vi "Weather_Client.vi"() -> ()   [LabVIEW 2024]
uses:
  <vilib>/express/express arith-compare/Formula/XNode/ExpressFormulaBlockNode.xnode
  <vilib>/httpClient/LabVIEWHTTPClient.lvlib
panel:
  in  "stop":bool
  out "Cloud Coverage [%]":dbl
  out "Slide":u8(slide) scale=0.0..100.0
  out "Wind Direction":dbl(knob) scale=0.0..312.0
  out "Wind Speed [m/s]":dbl(knob) scale=0.0..10.0
  out "Wind":T1
  out "Country":string
  out "Sunset (24h)":string
  out "Sunrise (24h)":string
  out "Current Time":timestamp format="%<%I:%M %p\n%x>T"
  out "Humidity Meter":dbl(knob) scale=0.0..100.0
  out "Humidity (%)":i32
  out "Pressure [hPa]":dbl
  out "Max Temp":dbl
  out "Min Temp":dbl
  out "Feels Like":dbl
  out "Thermometer":dbl(slide) scale=0.0..50.0
  in  "Select [°C/°F/K]":enum16{"Celcius", "Farenheit", "Kelvin"}(ring)
  out "Current Temp":dbl
  out "Status":cluster{"Sky":string, "Description":string}[](array[cluster])
  out "Coordinates":cluster{"Logitude":dbl, "Latitude":dbl}
  out "Visibility [km]":i32
  out "City Chosen":string
  in  "Enter City Name":string
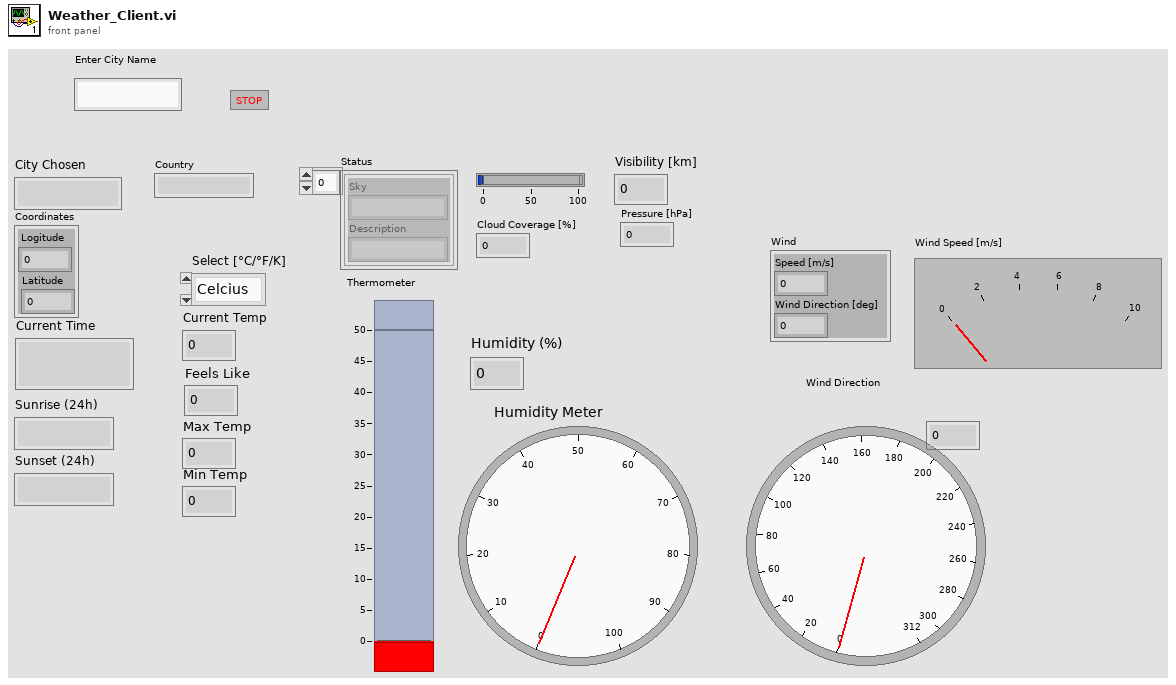
[diagram p1: front panel]
types:
  T1 = cluster{"Speed [m/s]":dbl, "Wind Direction [deg]":dbl}
  T2 = cluster{"sunrise":dbl, "sunset":dbl, "country":string}
  T3 = cluster{"temp":dbl, "feels_like":dbl, "temp_min":dbl, "temp_max":dbl, "pressure":dbl, "humidity":dbl}
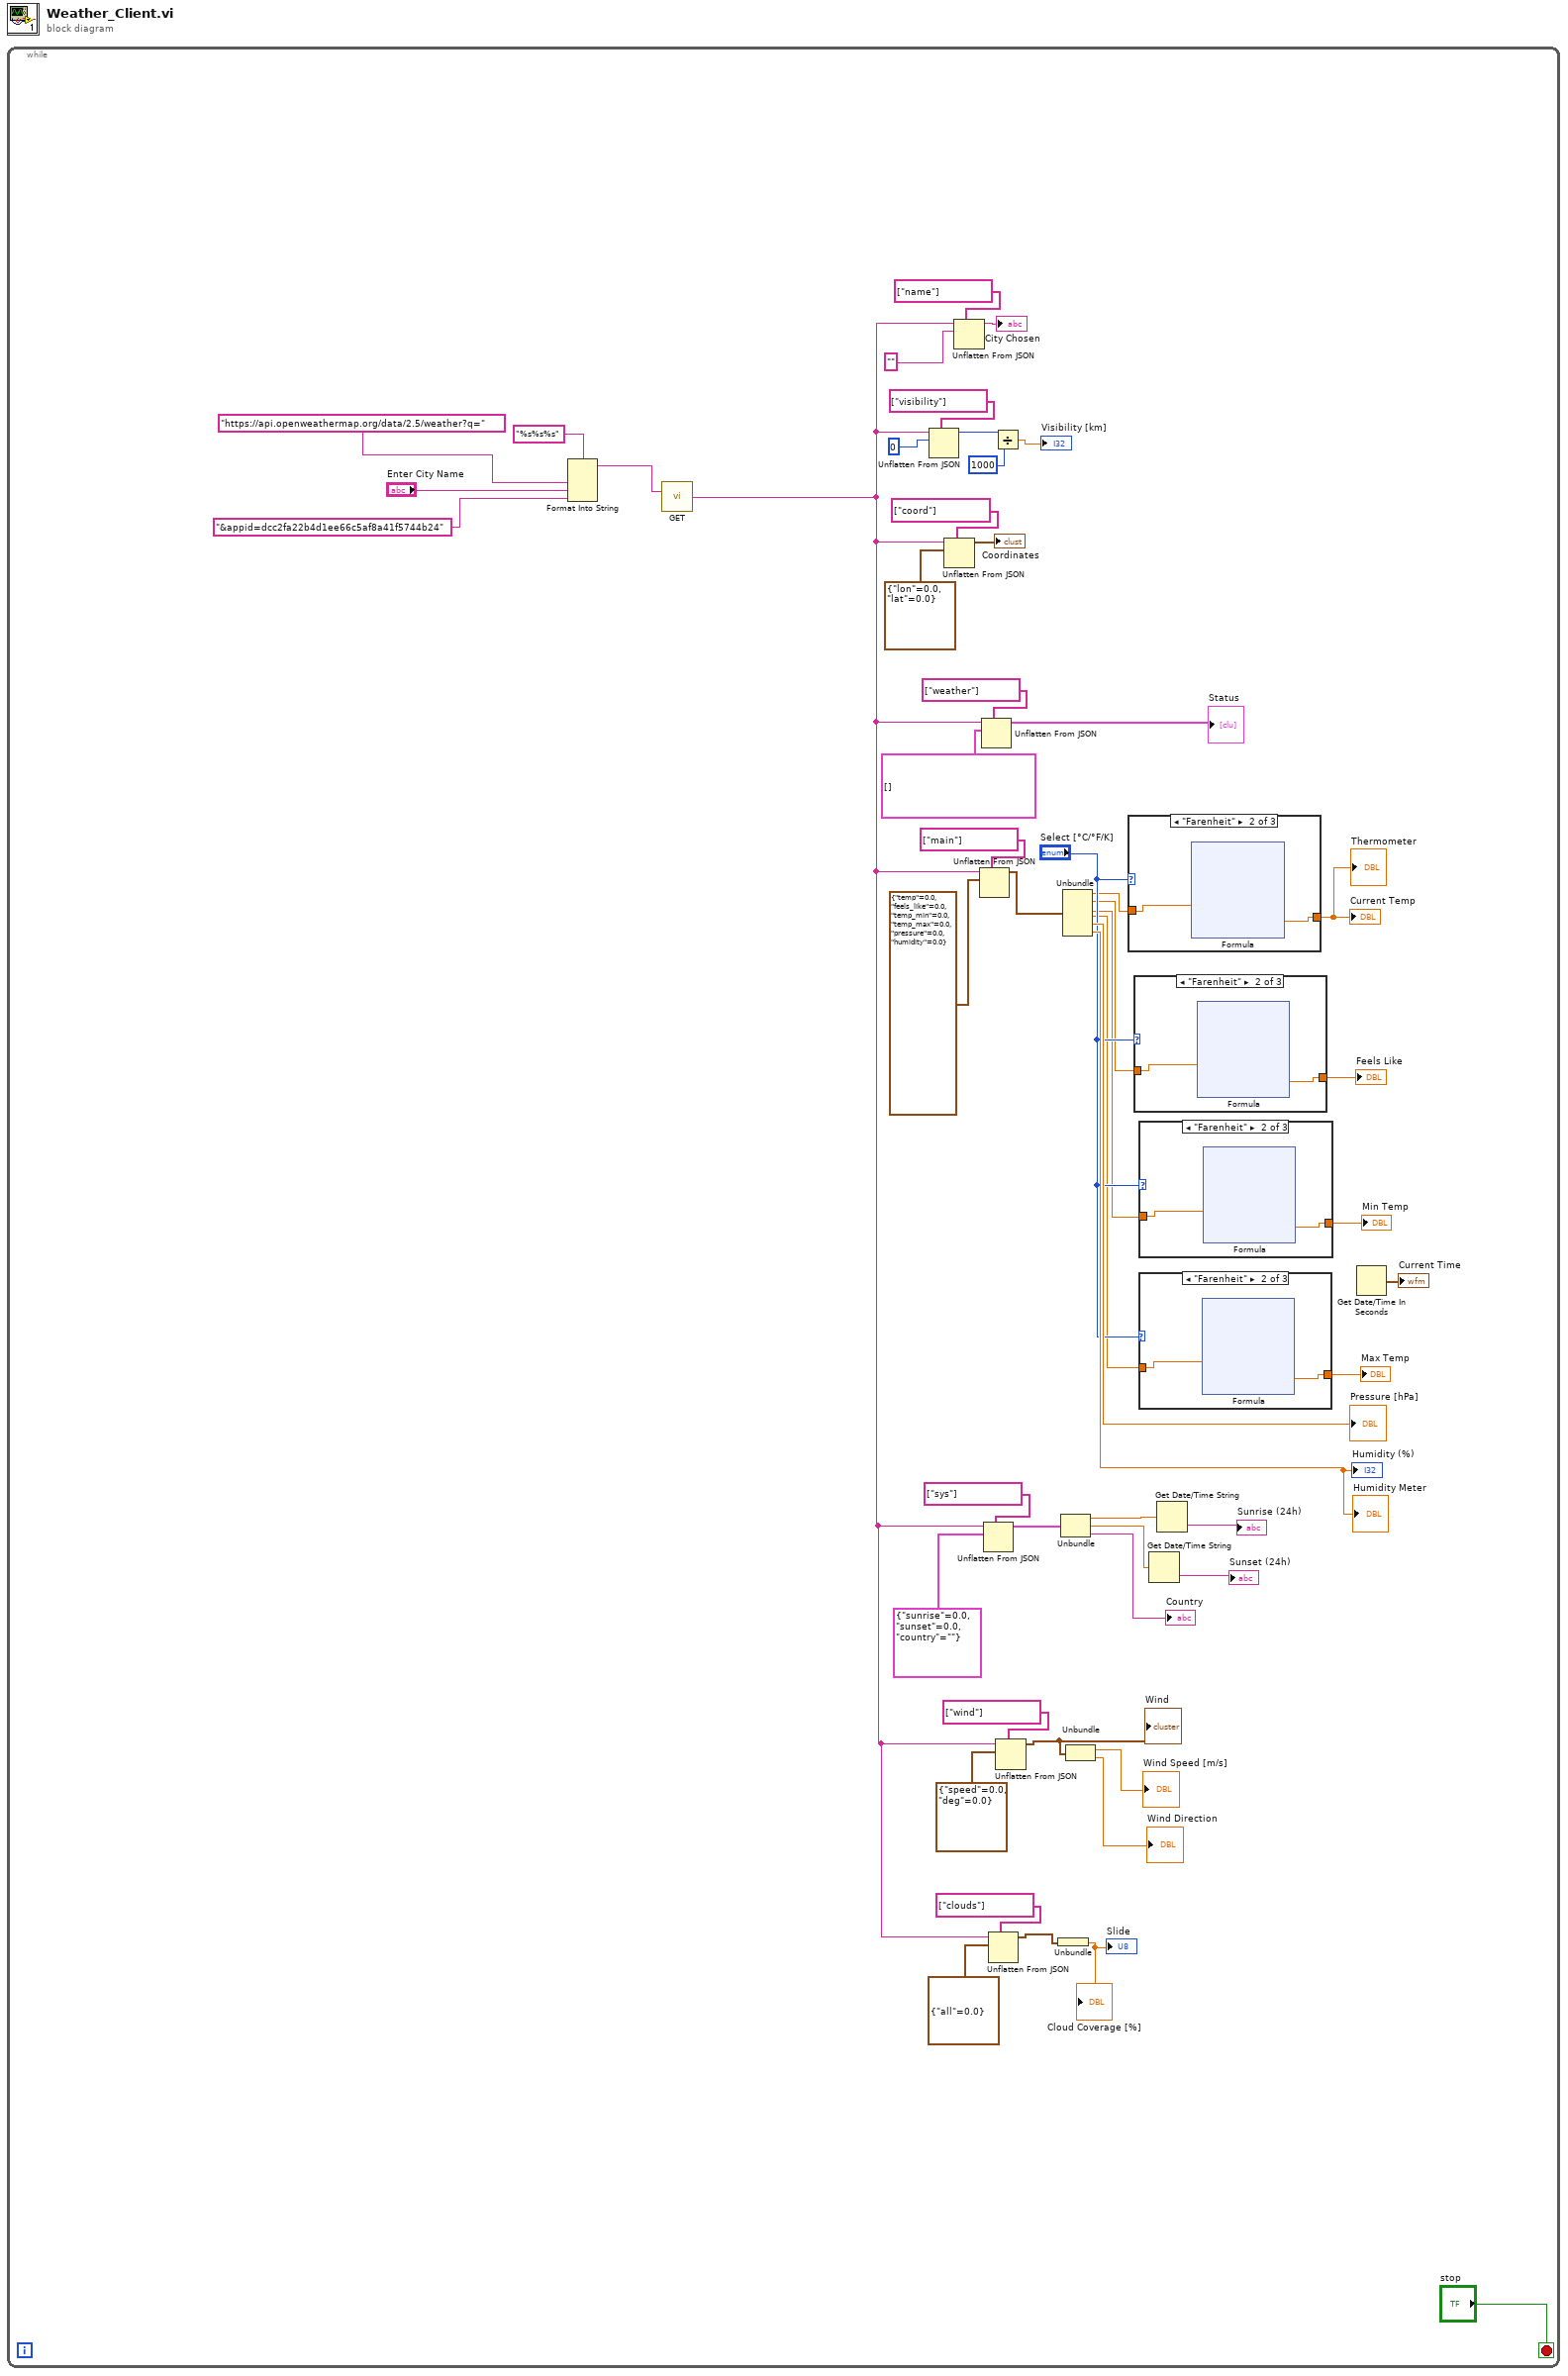
[diagram p0: block diagram]
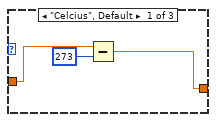
[diagram p2: hidden frame]
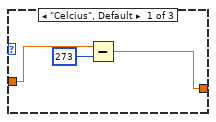
[diagram p4: hidden frame]
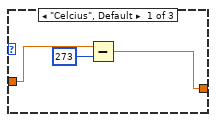
[diagram p6: hidden frame]
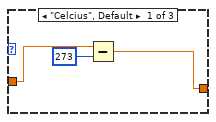
[diagram p8: hidden frame]
diagram:
  n1 = while {
    stop <- "stop" stop-if-true
    n2 = Format Into String(format string="%s%s%s", "https://api.openweathermap.org/data/2.5/weather?q=" ("input 1"), "Enter City Name", "&appid=dcc2fa22b4d1ee66c5af8a41f5744b24" ("input 3")) -> (resulting string=w22:string)  [unwired: 2 in, 1 out]
    n3 = call <vilib>:"GET.vi"("url"=w22) -> ("body"=w50:string)  [unwired: 11 in, 3 out]
    n4 = Unflatten From JSON(path=string[] ["visibility"], JSON string=w50, type and defaults=0 ("y")) -> (value=w24:i32)  [unwired: 4 in, 1 out]
    n5 = Unflatten From JSON(path=string[] ["coord"], JSON string=w50, type and defaults=cluster{"lon":dbl, "lat":dbl} {"lon"=0.0, "lat"=0.0}) -> (value=→"Coordinates":cluster{"lon":dbl, "lat":dbl})  [unwired: 4 in, 1 out]
    n6 = Unflatten From JSON(path=string[] ["name"], JSON string=w50, type and defaults="") -> (value=→"City Chosen":string)  [unwired: 4 in, 1 out]
    n7 = Unflatten From JSON(path=string[] ["main"], JSON string=w50, type and defaults=T3 {"temp"=0.0, "feels_like"=0.0, "temp_min"=0.0, "temp_max"=0.0, "pressure"=0.0, "humidity"=0.0}) -> (value=w30:T3)  [unwired: 4 in, 1 out]
    n8 = Unflatten From JSON(path=string[] ["weather"], JSON string=w50, type and defaults=cluster{"main":string, "description":string}[] []) -> (value=→"Status":cluster{"main":string, "description":string}[])  [unwired: 4 in, 1 out]
    n9 = Unflatten From JSON(path=string[] ["sys"], JSON string=w50, type and defaults=T2 {"sunrise"=0.0, "sunset"=0.0, "country"=""}) -> (value=w41:T2)  [unwired: 4 in, 1 out]
    n10 = Unflatten From JSON(path=string[] ["clouds"], JSON string=w50, type and defaults=cluster{"all":dbl} {"all"=0.0}) -> (value=w51:cluster{"all":dbl})  [unwired: 4 in, 1 out]
    n11 = Divide(x=w24, y=1000) -> (x/y=→"Visibility [km]":dbl)
    n12 = Unflatten From JSON(path=string[] ["wind"], JSON string=w50, type and defaults=cluster{"speed":dbl, "deg":dbl} {"speed"=0.0, "deg"=0.0}) -> (value=w47:cluster{"speed":dbl, "deg":dbl})  [unwired: 4 in, 1 out]
    "Wind" <- w47
    n13 = Unbundle(w51) -> ("all"=→"Slide" →"Cloud Coverage [%]":dbl)
    n14 = Unbundle(w41) -> ("sunrise"=w44:dbl, "sunset"=w45:dbl, "country"=→"Country":string)
    n15 = Unbundle(w30) -> ("temp"=w29:dbl, "feels_like"=w32:dbl, "temp_min"=w34:dbl, "temp_max"=w36:dbl, "pressure"=→"Pressure [hPa]":dbl, "humidity"=→"Humidity (%)" →"Humidity Meter":dbl)
    n16 = Unbundle(w47) -> ("speed"=→"Wind Speed [m/s]":dbl, "deg"=→"Wind Direction":dbl)
    n17 = case shown="\"Farenheit\"" "Select [°C/°F/K]" {
      tunnel: [w96 w99 w109] -> w28
      tunnel: w29 -> [w98 w100 w109]
      frame "Celcius", Default {
        n18 = Subtract(x=w98, y=273) -> (x-y=w96:dbl)
      }
      frame "Farenheit" {
        n19 = xnode "Formula"("X1"=w100) -> ("Result"=w99:dbl)  [unwired: 1 in, 1 out]
      }
      frame "Kelvin" {
      }
    }
    "Current Temp" <- w28
    "Thermometer" <- w28
    n20 = case shown="\"Farenheit\"" "Select [°C/°F/K]" {
      tunnel: [w82 w85 w95] -> w31
      tunnel: w32 -> [w84 w86 w95]
      frame "Celcius", Default {
        n21 = Subtract(x=w84, y=273) -> (x-y=w82:dbl)
      }
      frame "Farenheit" {
        n22 = xnode "Formula"("X1"=w86) -> ("Result"=w85:dbl)  [unwired: 1 in, 1 out]
      }
      frame "Kelvin" {
      }
    }
    "Feels Like" <- w31
    n23 = case shown="\"Farenheit\"" "Select [°C/°F/K]" {
      tunnel: [w54 w57 w67] -> w35
      tunnel: w36 -> [w56 w58 w67]
      frame "Celcius", Default {
        n24 = Subtract(x=w56, y=273) -> (x-y=w54:dbl)
      }
      frame "Farenheit" {
        n25 = xnode "Formula"("X1"=w58) -> ("Result"=w57:dbl)  [unwired: 1 in, 1 out]
      }
      frame "Kelvin" {
      }
    }
    "Max Temp" <- w35
    n26 = case shown="\"Farenheit\"" "Select [°C/°F/K]" {
      tunnel: [w68 w71 w81] -> w33
      tunnel: w34 -> [w70 w72 w81]
      frame "Celcius", Default {
        n27 = Subtract(x=w70, y=273) -> (x-y=w68:dbl)
      }
      frame "Farenheit" {
        n28 = xnode "Formula"("X1"=w72) -> ("Result"=w71:dbl)  [unwired: 1 in, 1 out]
      }
      frame "Kelvin" {
      }
    }
    "Min Temp" <- w33
    n29 = Get Date/Time String(seconds (now)=w45) -> (time string=→"Sunset (24h)":string)  [unwired: 2 in, 1 out]
    n30 = Get Date/Time String(seconds (now)=w44) -> (time string=→"Sunrise (24h)":string)  [unwired: 2 in, 1 out]
    n31 = Get Date/Time In Seconds() -> (seconds since 1Jan1904=→"Current Time":timestamp)
  }
